vi "test_Find Local Chassis Returns Ordered Modules.vi"(8 "error in (no error)":errorcluster, 11 "TestCase in":refnum<class "Scan Engine Scripting API Custom Device Unit Tests.lvclass">) -> (0 "error out":errorcluster, 3 "TestCase out":refnum<class "Scan Engine Scripting API Custom Device Unit Tests.lvclass">)   [LabVIEW 2019, in "Scan Engine Scripting API Custom Device Unit Tests.lvclass"]
uses:
  Scan Engine Scripting API Custom Device Unit Tests.lvclass
  <vilib>/addons/_JKI Toolkits/VI Tester/TestCase.llb/TestCase.lvclass
  Scripting/Scan Engine Scripting.lvlib
  Shared/Type Defs/Main Settings.ctl
  Shared/SEECD Shared.lvlib
  Shared/Type Defs/Local Chassis Settings.ctl
  Scripting/Modules/NI 9482/NI 9482.lvclass
  C:/Users/nitest/Desktop/Git 2019/niveristand-scan-engine-ethercat-custom-device/Custom Device Source/Scripting/Modules/Module/Module.lvclass
  C:/Program Files (x86)/National Instruments/LabVIEW 2019/vi.lib/addons/_JKI Toolkits/VI Tester/TestCase.llb/TestCase.lvclass
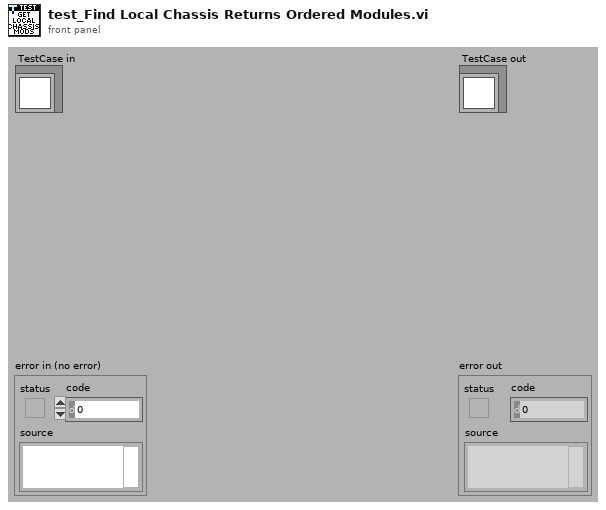
[diagram p1: front panel]
types:
  T1 = typedef "SEECD Shared.lvlib/Local Chassis Settings.ctl" = cluster{"name":string, "number of slots":i32}
  T2 = typedef "SEECD Shared.lvlib/Main Settings.ctl" = cluster{"sync to scan":bool, "scan engine decimation":u16, "delay after FPGA load (s)":u16}
  T3 = typedef "Custom Device API.lvlib/Custom Device Item Ref.ctl" = u64
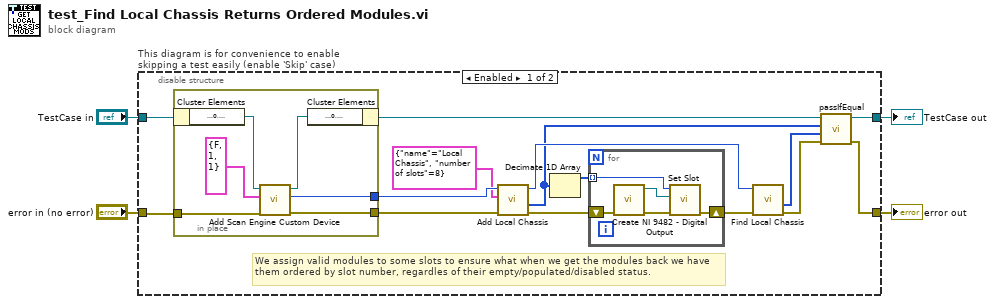
[diagram p0: block diagram]
diagram:
  n1 = disable-structure "This diagram is for convenience to enable skipping a test easily (enable 'Skip' case)" shown="Enabled" {
    disable-tunnel: "TestCase in" -> [w14 w34]
    disable-tunnel: [w15 w32] -> w1
    disable-tunnel: [w19 w33] -> w3
    disable-tunnel: "error in (no error)" -> [w16 w31]
    frame Enabled {
      # "We assign valid modules to some slots to ensure what when we get the modules back we have them ordered by slot number, regardles of their empty/populated/disabled status."
      n2 = in-place {
        in-place-border: [w25] -> w18
        in-place-border: [w24] -> w17
        in-place-border: w16 -> [w22]
        n3 = in-place-cluster #1(w14) -> ("target ref"=w21:refnum<k24>)
        n4 = call "Add Scan Engine Custom Device.vi"("error in"=w22, "settings"=T2 {"sync to scan"=FALSE, "scan engine decimation"=1, "delay after FPGA load (s)"=1}, "target in"=w21) -> ("error out"=w24:errorcluster, "scan engine custom device ref"=w25:T3, "target out"=w20:refnum<k24>)  [unwired: 6 in]
        n5 = in-place-cluster #1("target ref"=w20) -> (w13:refnum<class "Scan Engine Scripting API Custom Device Unit Tests.lvclass">)
      }
      n6 = call "Add Local Chassis.vi"("error in"=w17, "settings"=T1 {"name"="Local Chassis", "number of slots"=8}, "scan engine custom device ref in"=w18) -> ("error out"=w7:errorcluster, "slot refs"=w8:T3[], "scan engine custom device ref out"=w12:T3)  [unwired: 4 in, 2 out]
      n7 = Decimate 1D Array(w8) -> (w5:T3[])  [unwired: 2 out]
      n8 = for {
        tunnel: w5 -> [w26] mode=indexing
        shift-right: [w27] -> w6
        shift-left: w7 -> [w29]
        n9 = call "Create NI 9482 - Digital Output.vi"("error in"=w29) -> ("error out"=w28:errorcluster, "NI 9482 out"=w30:refnum<class "NI 9482.lvclass">)  [unwired: 9 in]
        n10 = call "Set Slot.vi"("error in"=w28, "module"=w30, "slot ref in"=w26) -> ("error out"=w27:errorcluster)  [unwired: 7 in, 1 out]
      }
      n11 = call "Find Local Chassis.vi"("error in"=w6, "scan engine custom device ref in"=w12) -> ("error out"=w10:errorcluster, "slots refs"=w11:T3[])  [unwired: 4 in, 4 out]
      n12 = call-dynamic "passIfEqual.vi"("error in (no error)"=w10, "y"=w11, "x"=w8, "TestCase in"=w13) -> ("error out"=w19:errorcluster, "TestCase out"=w15:refnum<class "Scan Engine Scripting API Custom Device Unit Tests.lvclass">)  [unwired: 6 in]
    }
    frame Disabled {
      # "skip test result while test is under development"
      n13 = call <vilib>:"skip.vi"("error in (no error)"=w31, "TestCase in"=w34) -> ("error out"=w33:errorcluster, "TestCase out"=w32:refnum<class "Scan Engine Scripting API Custom Device Unit Tests.lvclass">)  [unwired: 8 in]
    }
  }
  "error out" <- w3
  "TestCase out" <- w1
